vi "measure.vi"(8 "error in (no error)":errorcluster, 11 "Measurement in":refnum<class "Measurement.lvclass">) -> (0 "error out":errorcluster, 2 "result":refnum<class "MeasurementDatalvclass.lvclass">, 3 "Measurement out":refnum<class "Measurement.lvclass">)   [LabVIEW 2017, in "Measurement.lvclass"]
doc: "Do measure"
uses:
  Measurement.lvclass
  measurement_data/MeasurementDatalvclass.lvclass
  Measurement.lvclass/Measurement.ctl
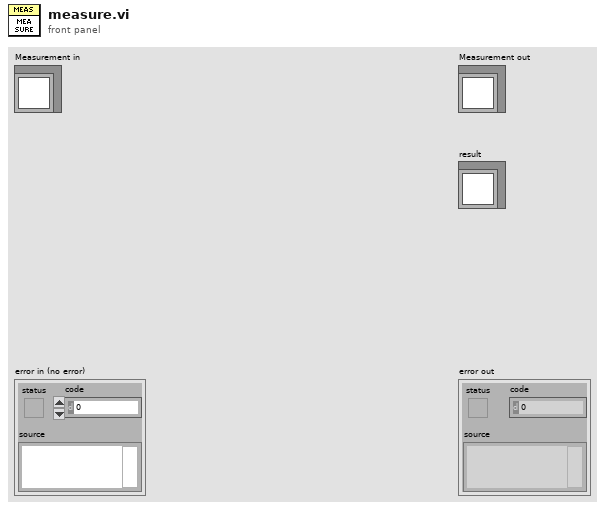
[diagram p1: front panel]
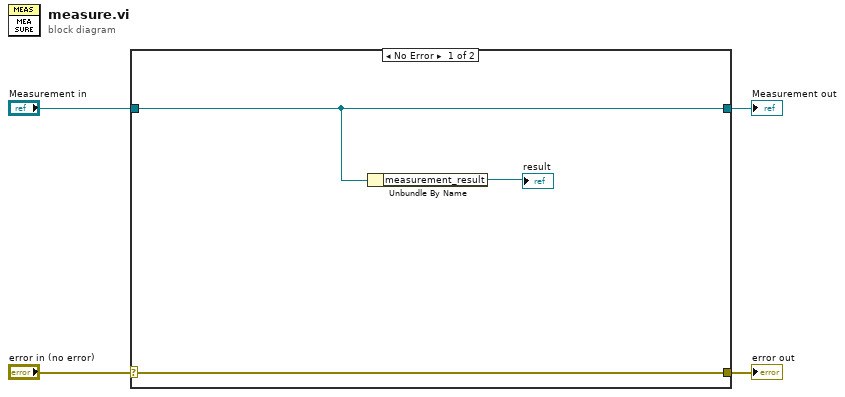
[diagram p0: block diagram]
diagram:
  n1 = case shown="No Error" "error in (no error)" {
    selector: "error in (no error)" -> [w7 w9]
    tunnel: [w7 w9] -> w3
    tunnel: [w6 w8] -> w1
    tunnel: "Measurement in" -> [w6 w8]
    frame No Error {
      n2 = Unbundle By Name(w6) -> ("measurement_result"=→"result":refnum<class "MeasurementDatalvclass.lvclass">)
    }
    frame Error {
    }
  }
  "error out" <- w3
  "Measurement out" <- w1
